vi "Build.vi"   [LabVIEW 2020, in "NI_App_Builder_API.lvlib"]
doc: "Builds a build specification using the properties in memory that you configure when you right-click a build specification and select <B>Properties</B>. To use this VI, you previously configure the build specification using the <B>Properties</B> shortcut menu option."
uses:
  <vilib>/AppBuilder/AB_API_Simple/NI_App_Builder_API.lvlib
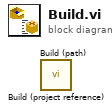
[diagram p0: block diagram]
diagram:
  n1 = call <vilib>:"Build (project reference).vi"() -> ()  [unwired: 9 in, 3 out]
  n2 = call <vilib>:"Build (path).vi"() -> ()  [unwired: 10 in, 2 out]
